vi "testpair client.vi"() -> ()   [LabVIEW 2016]
uses:
  dllwrapper/action complete event.ctl
  tls classes/connection creator/client connector/client connector.lvclass
  C:/Users/IEUser/Desktop/libasynclvtls/tls classes/connection creator/connection creator.lvclass
  tls classes/engine context/engine context.lvclass
  tls classes/connection/connection.lvclass
  tls classes/connection creator/connection creator.lvclass
  dllwrapper/async tls dl.lvlib
panel:
  out "dt":dbl
  in  "send all":bool
  in  "pull data":bool
  out "remaining data":string
  out "read bytes":i32
  out "write bytes":i32
  in  "read":bool
  in  "send":bool
  in  "stop":bool
  out "error out":errorcluster
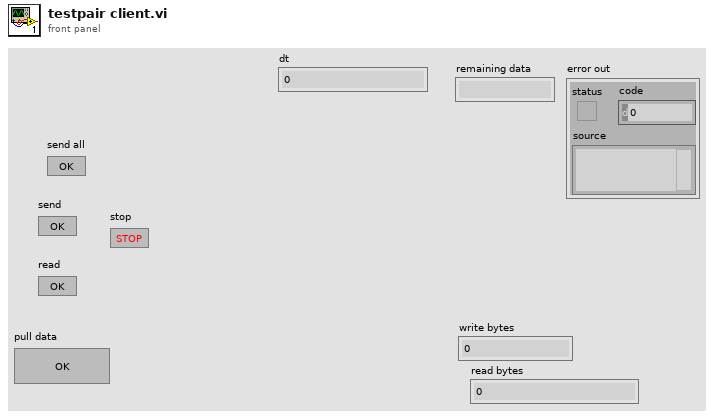
[diagram p1: front panel]
types:
  T1 = typedef "async tls dl.lvlib/action complete event.ctl" = cluster{"request ID":u32, "error code":i32, "error string":string}
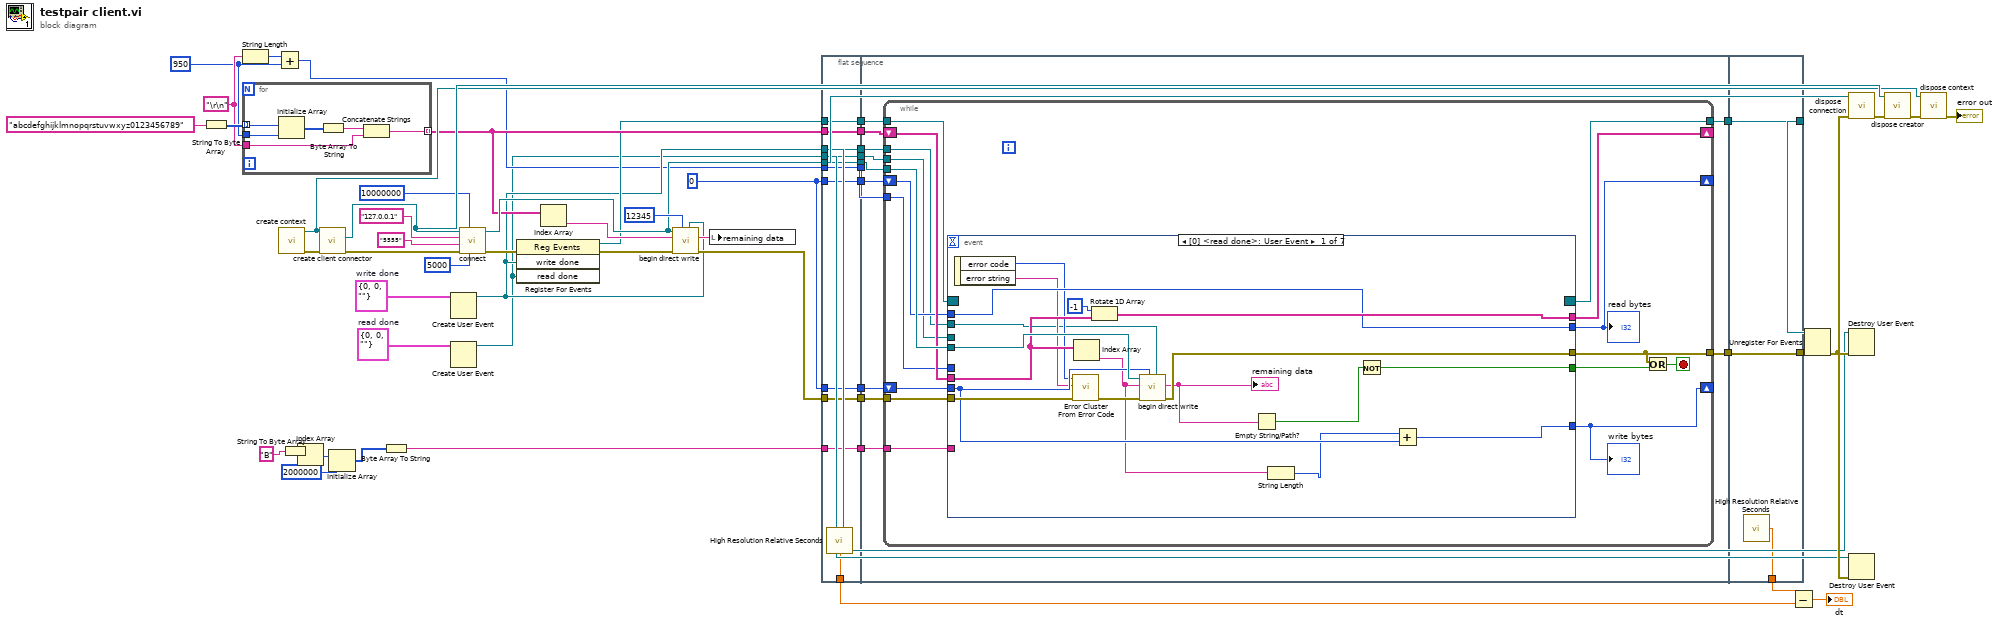
[diagram p0: block diagram]
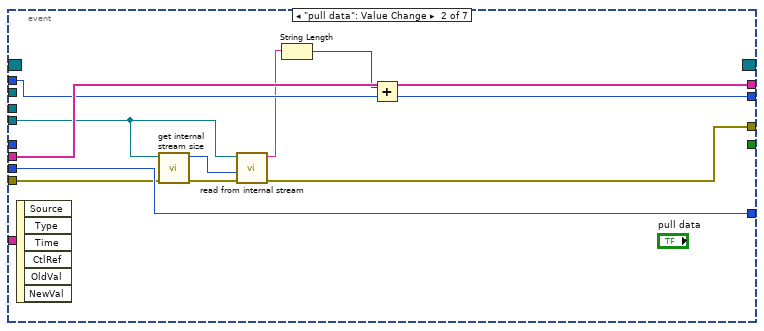
[diagram p2: hidden frame]
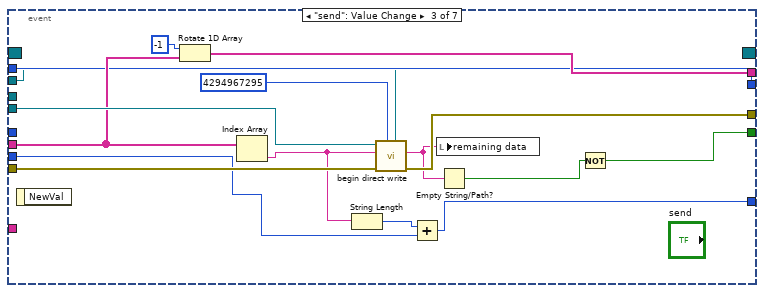
[diagram p3: hidden frame]
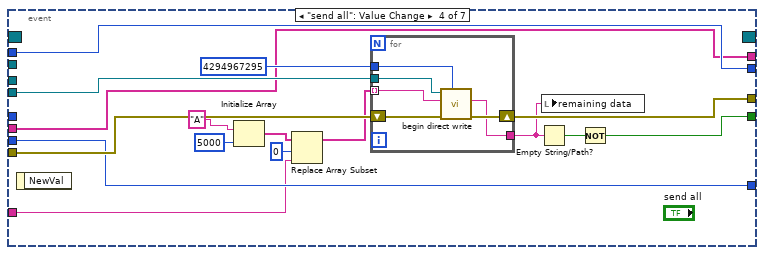
[diagram p4: hidden frame]
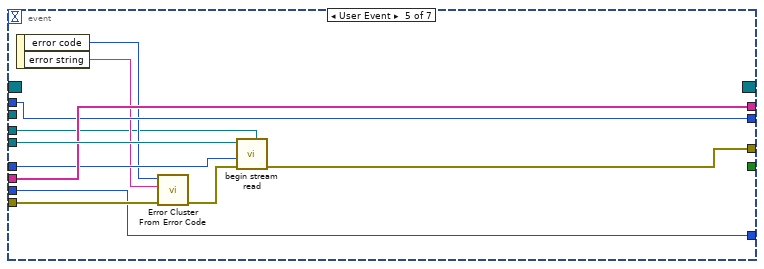
[diagram p5: hidden frame]
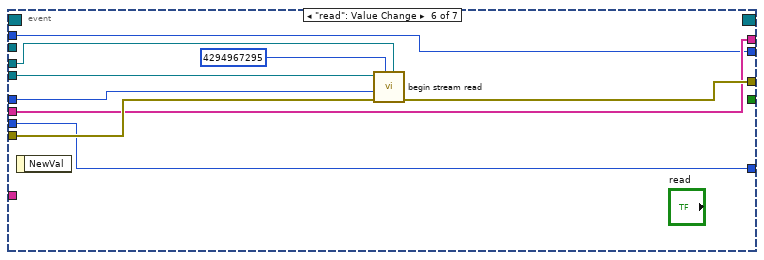
[diagram p6: hidden frame]
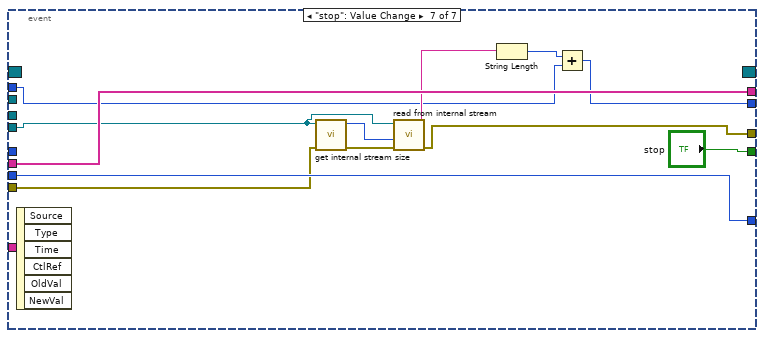
[diagram p7: hidden frame]
diagram:
  w32 = T1 {"request ID"=0, "error code"=0, "error string"=""}  # read done
  w33 = T1 {"request ID"=0, "error code"=0, "error string"=""}  # write done
  w35 = "\r\n" ("termination")
  w36 = 0
  w22 = 950 ("dimension size")
  n1 = String To Byte Array(string="abcdefghijklmnopqrstuvwxyz0123456789") -> (unsigned byte array=w40:u8[])
  n2 = String Length(string=w35) -> (length=w34:i32)
  n3 = for {
    tunnel: w40 -> [w61] mode=indexing
    tunnel: [w58] -> w39 mode=indexing
    tunnel: w35 -> [w57]
    tunnel: w22 -> [w56]
    n4 = Initialize Array(w61, w56) -> (w60:u8[])
    n5 = Byte Array To String(unsigned byte array=w60) -> (string=w59:string)
    n6 = Concatenate Strings(w59, w57) -> (w58:string)
  }
  n7 = Add(x=w34, y=w22) -> (x+y=w25:i32)
  n8 = call "create context.vi"() -> ("error out"=w55:errorcluster, "engine context out"=w45:refnum<class "engine context.lvclass">)  [unwired: 10 in]
  n9 = String To Byte Array(string="B") -> (unsigned byte array=w20:u8[])
  n10 = Index Array(array=w20) -> (element=w18:u8)  [unwired: 1 in]
  n11 = call "create client connector.vi"("error in"=w55, "engine context in"=w45) -> ("error out"=w54:errorcluster, "client connector out"=w47:refnum<class "client connector.lvclass">)  [unwired: 8 in]
  n12 = Initialize Array(w18, 2000000 ("dimension size")) -> (w19:u8[])
  n13 = Byte Array To String(unsigned byte array=w19) -> (string=w16:string)
  n14 = Create User Event(user event datatype=w33) -> (user event=w26:refnum<user-event>)  [unwired: 1 in, 1 out]
  n15 = Create User Event(user event datatype=w32) -> (user event=w24:refnum<user-event>)  [unwired: 1 in, 1 out]
  n16 = call "connect.vi"("timeout"=5000, "stream buffer size"=u64 10000000, "error in"=w54, "port"="5555", "host"="127.0.0.1", "client connector in"=w47) -> ("error out"=w30:errorcluster, "connection out"=w43:refnum<class "connection.lvclass">)  [unwired: 4 in]
  n17 = register-events(error in=w30, w26, w24) -> (reference out=w28:refnum<event-registration>, error out=w29:errorcluster)  [unwired: 1 in]
  n18 = Index Array(array=w39) -> (element=w37:string)  [unwired: 1 in]
  n19 = call "begin direct write.vi"("event"=w26, "id"=u32 12345, "error in"=w29, "data"=w37, "connection in"=w43) -> ("error out"=w49:errorcluster, "remaining data"=w27:string)  [unwired: 5 in]
  n20 = local write "remaining data"(w27) -> ()
  n21 = flat-sequence {
    tunnel: w16 -> [w63]
    tunnel: w24 -> [w64]
    tunnel: w25 -> [w65]
    tunnel: w26 -> [w66]
    tunnel: w28 -> [w67]
    tunnel: w36 -> [w68]
    tunnel: w36 -> [w69]
    tunnel: w39 -> [w70]
    tunnel: w43 -> [w71]
    tunnel: w49 -> [w72]
    tunnel: [w72] -> w15
    tunnel: [w71] -> w14
    tunnel: [w70] -> w13
    tunnel: [w69] -> w12
    tunnel: [w68] -> w11
    tunnel: [w67] -> w10
    tunnel: [w66] -> w9
    tunnel: [w65] -> w8
    tunnel: [w64] -> w7
    tunnel: [w63] -> w6
    tunnel: [w62] -> w2
    tunnel: w15 -> [w84]
    tunnel: w14 -> [w83]
    tunnel: w13 -> [w80]
    tunnel: w12 -> [w79]
    tunnel: w11 -> [w78]
    tunnel: w10 -> [w77]
    tunnel: w9 -> [w76]
    tunnel: w8 -> [w75]
    tunnel: w7 -> [w74]
    tunnel: w6 -> [w73]
    tunnel: [w82] -> w5
    tunnel: [w81] -> w4
    tunnel: [w202] -> w41
    tunnel: [w203] -> w42
    tunnel: w5 -> [w203]
    tunnel: w4 -> [w202]
    tunnel: [w201] -> w3
    frame #0 {
      n22 = call <vilib>:"High Resolution Relative Seconds.vi"() -> ("relative seconds"=w62:dbl)
    }
    frame #1 {
      n23 = while {
        tunnel: w77 -> [w101]
        tunnel: w83 -> [w99]
        tunnel: [w95] -> w81
        shift-right: [w93] -> _
        shift-left: w80 -> [w94]
        tunnel: w75 -> [w92]
        tunnel: w84 -> [w100]
        tunnel: [w96] -> w82
        shift-right: [w90] -> _
        shift-left: w79 -> [w91]
        shift-right: [w89] -> _
        shift-left: w78 -> [w88]
        tunnel: w76 -> [w87]
        tunnel: w74 -> [w86]
        tunnel: w73 -> [w85]
        stop <- w97 stop-if-true
        n24 = event shown="[0] <read done>: User Event" {
          selector: w101 -> [_ _ _ _ _ _ _]
          dyn-events: [_ _ _ _ _ _ _] -> w95
          timeout: _ -> [_ _ _ _ _ _ _]
          tunnel: w100 -> [w119 w123 w146 w162 w179 w188 w194]
          tunnel: [w118 w126 w145 w161 w177 w186 w195] -> w96
          tunnel: w99 -> [w117 w125 w144 w160 w178 w187 w193]
          tunnel: [w105 _ w136 w155 _ _ "stop"] -> w98
          tunnel: w94 -> [w114 w130 w141 w153 w176 w185 w199]
          tunnel: [w116 w130 w142 w153 w176 w185 w199] -> w93
          tunnel: w92 -> [_ _ _ _ w173 w184 _]
          tunnel: w91 -> [w113 w129 w140 w159 w175 w183 w190]
          tunnel: [w113 w121 w140 w159 w175 w183 w189] -> w90
          tunnel: [w112 w128 w131 w158 w174 w182 w198] -> w89
          tunnel: w88 -> [w111 w128 w132 w158 w174 w182 w198]
          tunnel: w87 -> [w107 _ w139 _ _ _ _]
          tunnel: w86 -> [_ _ _ _ w169 w181 _]
          tunnel: w85 -> [_ _ _ w147 _ _ _]
          event User Event {
            n25 = event-data() -> ("error code"=w109:i32, "error string"=w108:string)  [unwired: 1 in]
            n26 = call <vilib>:"Error Cluster From Error Code.vi"("error in (no error)"=w119, "error message (\"\")"=w108, "error code (0)"=w109) -> ("error out"=w110:errorcluster)  [unwired: 6 in]
            n27 = Index Array(array=w114) -> (element=w103:string)  [unwired: 1 in]
            n28 = Rotate 1D Array(1:w114, 2:-1 ("n")) -> (0:w116:string[])
            n29 = call "begin direct write.vi"("event"=w107, "id"=w111, "error in"=w110, "data"=w103, "connection in"=w117) -> ("error out"=w118:errorcluster, "remaining data"=w104:string)  [unwired: 5 in]
            "remaining data" <- w104
            n30 = Empty String/Path?(string/path=w104) -> (empty?=w106:bool)
            n31 = String Length(string=w103) -> (length=w102:i32)
            n32 = Not(x=w106) -> (.not. x?=w105:bool)
            n33 = Add(x=w102, y=w111) -> (x+y=w112:i32)
          }
          event "pull data": Value Change {
            n34 = event-data() -> ()  [unwired: 1 in, 6 out]
            n35 = call "get internal stream size.vi"("error in"=w123, "connection in"=w125) -> ("error out"=w127:errorcluster, "size"=w124:u64)  [unwired: 8 in]
            n36 = call "read from internal stream.vi"("error in"=w127, "max length"=w124, "connection in"=w125) -> ("error out"=w126:errorcluster, "buffer"=w122:string)  [unwired: 7 in]
            n37 = String Length(string=w122) -> (length=w120:i32)
            n38 = Add(x=w120, y=w129) -> (x+y=w121:i32)
          }
          event "send": Value Change {
            n39 = event-data() -> ()  [unwired: 1 in, 1 out]
            n40 = Rotate 1D Array(1:w141, 2:-1 ("n")) -> (0:w142:string[])
            n41 = Index Array(array=w141) -> (element=w133:string)  [unwired: 1 in]
            n42 = String Length(string=w133) -> (length=w134:i32)
            n43 = call "begin direct write.vi"("event"=w139, "id"=u32 4294967295, "error in"=w146, "data"=w133, "connection in"=w144) -> ("error out"=w145:errorcluster, "remaining data"=w135:string)  [unwired: 5 in]
            n44 = Add(x=w134, y=w132) -> (x+y=w131:i32)
            n45 = local write "remaining data"(w135) -> ()
            n46 = Empty String/Path?(string/path=w135) -> (empty?=w137:bool)
            n47 = Not(x=w137) -> (.not. x?=w136:bool)
          }
          event "send all": Value Change {
            n48 = event-data() -> ()  [unwired: 1 in, 1 out]
            n49 = Initialize Array("A" ("termination"), 5000 ("dimension size")) -> (w150:string[])
            n50 = Replace Array Subset(array=w150, new element=w147, index=0) -> (w149:string[])
            n51 = for {
              tunnel: w160 -> [w166]
              tunnel: u32 4294967295 ("id") -> [w165]
              tunnel: [w164] -> w154
              shift-right: [w167] -> w161
              shift-left: w162 -> [w168]
              tunnel: w149 -> [w163] mode=indexing
              n52 = call "begin direct write.vi"("id"=w165, "error in"=w168, "data"=w163, "connection in"=w166) -> ("error out"=w167:errorcluster, "remaining data"=w164:string)  [unwired: 6 in]
            }
            n53 = Empty String/Path?(string/path=w154) -> (empty?=w156:bool)
            n54 = local write "remaining data"(w154) -> ()
            n55 = Not(x=w156) -> (.not. x?=w155:bool)
          }
          event User Event {
            n56 = event-data() -> ("error code"=w170:i32, "error string"=w171:string)  [unwired: 1 in]
            n57 = call <vilib>:"Error Cluster From Error Code.vi"("error in (no error)"=w179, "error message (\"\")"=w171, "error code (0)"=w170) -> ("error out"=w172:errorcluster)  [unwired: 6 in]
            n58 = call "begin stream read.vi"("event"=w169, "error in"=w172, "max bytes to read"=w173, "connection in"=w178) -> ("error out"=w177:errorcluster)  [unwired: 7 in]
          }
          event "read": Value Change {
            n59 = event-data() -> ()  [unwired: 1 in, 1 out]
            n60 = call "begin stream read.vi"("event"=w181, "id"=u32 4294967295, "error in"=w188, "max bytes to read"=w184, "connection in"=w187) -> ("error out"=w186:errorcluster)  [unwired: 6 in]
          }
          event "stop": Value Change {
            n61 = event-data() -> ()  [unwired: 1 in, 6 out]
            n62 = call "get internal stream size.vi"("error in"=w194, "connection in"=w193) -> ("error out"=w197:errorcluster, "size"=w196:u64)  [unwired: 8 in]
            n63 = call "read from internal stream.vi"("error in"=w197, "max length"=w196, "connection in"=w193) -> ("error out"=w195:errorcluster, "buffer"=w192:string)  [unwired: 7 in]
            n64 = String Length(string=w192) -> (length=w191:i32)
            n65 = Add(x=w191, y=w190) -> (x+y=w189:i32)
          }
        }
        "write bytes" <- w89
        "read bytes" <- w90
        n66 = Or(x=w96, y=w98) -> (x .or. y?=w97:bool)
      }
    }
    frame #2 {
      n67 = call <vilib>:"High Resolution Relative Seconds.vi"() -> ("relative seconds"=w201:dbl)
    }
  }
  n68 = Subtract(x=w3, y=w2) -> (x-y=→"dt":dbl)
  n69 = Unregister For Events(event registration refnum=w41, error in=w42) -> (error out=w31:errorcluster)
  n70 = call "dispose connection.vi"("error in"=w31, "connection in"=w43) -> ("error out"=w48:errorcluster)  [unwired: 9 in]
  n71 = Destroy User Event(user event=w26, error in=w31) -> ()  [unwired: 1 out]
  n72 = Destroy User Event(user event=w24, error in=w31) -> ()  [unwired: 1 out]
  n73 = call "dispose creator.vi"("error in"=w48, "connection creator in"=w47) -> ("error out"=w46:errorcluster)  [unwired: 9 in]
  n74 = call "dispose context.vi"("error in"=w46, "engine context out"=w45) -> ("error out"=→"error out":errorcluster)  [unwired: 9 in]
